vi "sequencerReadTracks.vi"(10 "nOfScanRegions":i32) -> (1 "arrayOfTracks":i32[](array[numeric]))   [LabVIEW 2014]
uses:
  <vilib>/rvi/Emulation/niFpgaSctlEmulationGetInTimedLoop.vi
  sequencerGlobVars.vi
  <vilib>/rvi/Emulation/niFpgaProcessEmulError.vi
  <vilib>/rvi/interface/RandomDataEmulation/niFpgaRandomDataHandleErrors.vi
  <vilib>/rvi/DataTransferAndStorage/Container/XNode/niFpgaContainer.xnode
  <vilib>/rvi/interface/RandomDataEmulation/nirviRandomDataFpgaReadWriteTemplate.vi
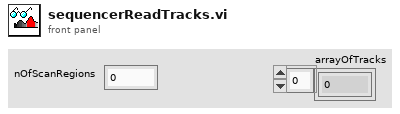
[diagram p1: front panel]
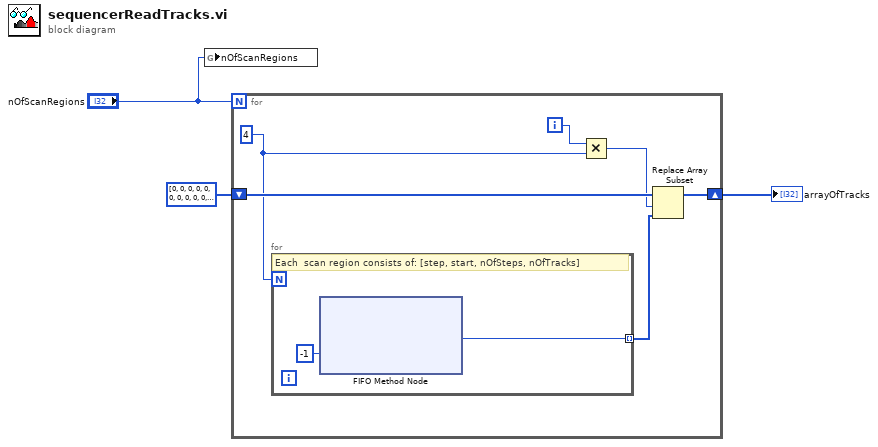
[diagram p0: block diagram]
diagram:
  n1 = global write "sequencerGlobVars.vi" "nOfScanRegions"("nOfScanRegions") -> ()
  n2 = for {
    N: "nOfScanRegions" -> [_]
    shift-right: [w8] -> w2
    shift-left: i32[] [0, 0, 0, 0, 0, 0, 0, 0, 0, 0, 0, 0, 0, 0, 0, 0, 0, 0, 0, 0, 0, 0, 0, 0, 0, 0, 0, 0, 0, 0, 0, 0, 0, 0, 0, 0, 0, 0, 0, 0, 0, 0, 0, 0, 0, 0, 0, 0, 0, 0, 0, 0, 0, 0, 0, 0, 0, 0, 0, 0, 0, 0, 0, 0, 0, 0, 0, 0, 0] -> [w9]
    i -> [w6]
    w5 = 4 ("y")
    n3 = for {
      N: w5 -> [_]
      tunnel: [w11] -> w7 mode=indexing
      # "Each  scan region consists of: [step, start, nOfSteps, nOfTracks]"
      n4 = xnode ("FIFO Method Node")("Timeout"=-1) -> ("Element"=w11:i32)  [unwired: 1 in, 2 out]
    }
    n5 = Multiply(x=w6, y=w5) -> (x*y=w4:i32)
    n6 = Replace Array Subset(array=w9, new element=w7, index=w4) -> (w8:i32[])
  }
  "arrayOfTracks" <- w2
